vi "Handle Request.vi"(7 "Processing In":refnum<class "Processing.lvclass">, 11 "Request Session Handler in":refnum<class "Request Session Handler.lvclass">) -> (0 "error out":errorcluster, 5 "Processing":refnum<class "Processing.lvclass">)   [LabVIEW 2020, in "HTTP Server.lvlib" / "Request Session Handler.lvclass"]
uses:
  Request Session Handler.lvclass
  Processing/Processing.lvclass
  Processing/Processing.lvclass/Processing.ctl
  lv-http-util/HTTP Utils/Request/Request.lvclass
  Session/Session.lvclass
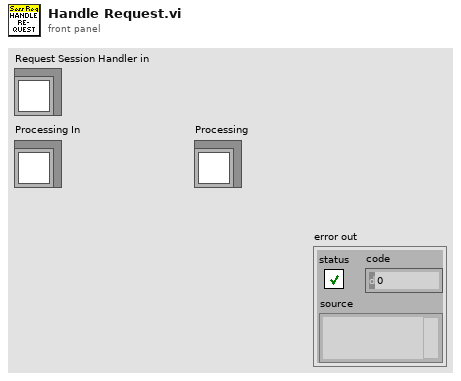
[diagram p1: front panel]
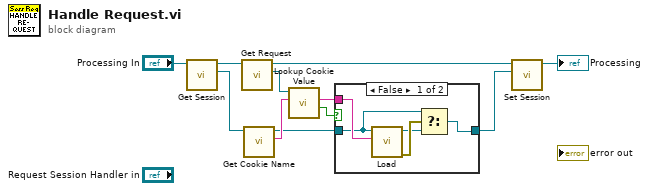
[diagram p0: block diagram]
diagram:
  n1 = call "Get Session.vi"("Processing in"="Processing In") -> ("Session"=w6:refnum<class "Session.lvclass">, "Processing out"=w4:refnum<class "Processing.lvclass">)  [unwired: 9 in]
  n2 = call "Get Request.vi"("Processing in"=w4) -> ("Request"=w5:refnum<class "Request.lvclass">, "Processing out"=w3:refnum<class "Processing.lvclass">)  [unwired: 9 in]
  n3 = call "Get Cookie Name.vi"("Session in"=w6) -> ("Cookie Name"=w11:string, "Session out"=w10:refnum<class "Session.lvclass">)  [unwired: 8 in, 1 out]
  n4 = call "Lookup Cookie Value.vi"("Name"=w11, "Request in"=w5) -> ("Not Found?"=w8:bool, "Value"=w9:string)  [unwired: 6 in, 2 out]
  n5 = case shown="False" w8 {
    tunnel: w10 -> [w13 w17]
    tunnel: w9 -> [w16 _]
    tunnel: [w12 w17] -> w2
    frame False {
      n6 = call "Load.vi"("ID"=w16, "Session in"=w13) -> ("error out"=w15:errorcluster, "Session out"=w14:refnum<class "Session.lvclass">)  [unwired: 8 in]
      n7 = Select(t=w13, s=w15, f=w14) -> (s? t:f=w12:refnum<class "Session.lvclass">)
    }
    frame True {
    }
  }
  n8 = call "Set Session.vi"("Session"=w2, "Processing in"=w3) -> ("Processing out"=→"Processing":refnum<class "Processing.lvclass">)  [unwired: 9 in]
